vi "Open UI.vi"(8 "error in (no error)":errorcluster, 11 "Process in":refnum<class "Process.lvclass">) -> (0 "error out":errorcluster, 3 "Process out":refnum<class "Process.lvclass">)   [LabVIEW 2021, in "Process.lvlib" / "Process.lvclass"]
uses:
  Process.lvclass
  Process.lvclass/Process.ctl
  LVCAM/Msgs/LVCAM Destroy Self/LVCAM Destroy Self Msg/LVCAM Destroy Self Msg.lvclass
  C:/PPLs/LabVIEW-Composed-Actor-Model-LVCAM/LabVIEW-Composed-Actor-Model-LVCAM/LVCAM/LVCAM/Msg/Msg.lvclass
  LVCAM/LVCAM/Self Actor/Self Msg Send.vi
  LVCAM/LVCAM/Self Actor/Self Actor.lvclass
  C:/PPLs/LabVIEW-Composed-Actor-Model-LVCAM/LabVIEW-Composed-Actor-Model-LVCAM/LVCAM/Msgs/LVCAM Destroy Self/LVCAM Destroy Self Msg/LVCAM Destroy Self Msg.lvclass
  C:/PPLs/LabVIEW-Composed-Actor-Model-LVCAM/LabVIEW-Composed-Actor-Model-LVCAM/LVCAM/Msgs/LVCAM Destroy Self/LVCAM Destroy Self/LVCAM Destroy Self.lvclass
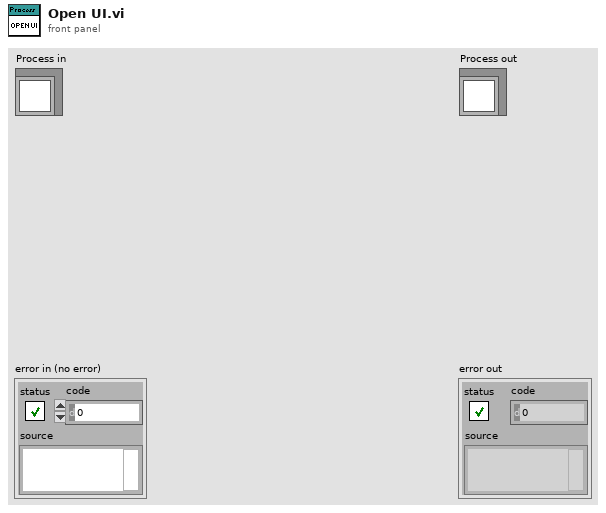
[diagram p1: front panel]
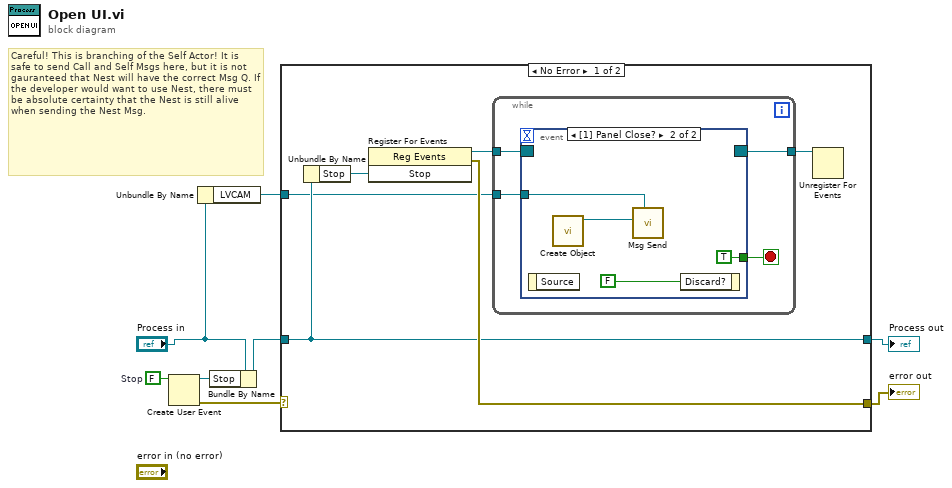
[diagram p0: block diagram]
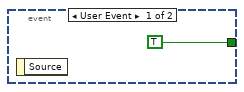
[diagram p2: hidden frame]
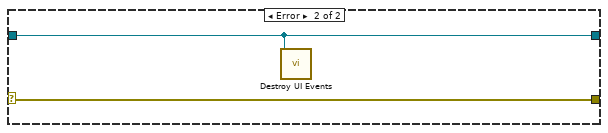
[diagram p3: hidden frame]
diagram:
  w7 = FALSE  # Stop
  # "Careful! This is branching of the Self Actor! It is safe to send Call and Self Msgs here, but it is not gauranteed that Nest will have the correct Msg Q. If the developer would want to use Nest, there must be absolute certainty that the Nest is still alive when sending the Nest Msg."
  n1 = Create User Event(user event datatype=w7) -> (user event=w8:refnum<user-event>, error out=w6:errorcluster)  [unwired: 1 in]
  n2 = Unbundle By Name("Process in") -> ("LVCAM"=w5:refnum<class "LVCAM.lvclass">)
  n3 = Bundle By Name(cluster="Process in", "Stop"=w8) -> (w4:refnum<class "Process.lvclass">)
  n4 = case shown="No Error" w6 {
    selector: w6 -> [_ w25]
    tunnel: [w12 w25] -> w3
    tunnel: w4 -> [w10 w24]
    tunnel: [w10 w24] -> w1
    tunnel: w5 -> [w9 _]
    frame No Error {
      n5 = Unbundle By Name(w10) -> ("Stop"=w11:refnum<user-event>)
      n6 = register-events ("Main Register for Events")(w11) -> (reference out=w14:refnum<event-registration>, error out=w12:errorcluster)  [unwired: 2 in]
      n7 = while {
        tunnel: w14 -> [w18]
        tunnel: [w16] -> w13
        tunnel: w9 -> [w15]
        stop <- w17 stop-if-true
        n8 = event "UI Events" shown="[1] Panel Close?" {
          selector: w18 -> [_ _]
          dyn-events: [_ _] -> w16
          timeout: _ -> [_ _]
          tunnel: [TRUE TRUE] -> w17
          tunnel: w15 -> [_ w23]
          event User Event {
            n9 = event-data() -> ()  [unwired: 1 in, 1 out]
          }
          event Panel Close? {
            n10 = event-data() -> ()  [unwired: 1 in, 1 out]
            n11 = call "Create Object.vi"() -> ("LVCAM Destroy Self Msg out"=w22:refnum<class "LVCAM Destroy Self Msg.lvclass">)  [unwired: 11 in]
            n12 = call-poly "Msg Send.vi"("Self Actor"=w23, "Msg"=w22) -> ()  [unwired: 9 in, 1 out]
            n13 = event-data("Discard?"=FALSE) -> ()  [unwired: 1 in, 1 out]
          }
        }
      }
      n14 = Unregister For Events(event registration refnum=w13) -> ()  [unwired: 1 in, 1 out]
    }
    frame Error {
      n15 = call "Destroy UI Events.vi"("Process in"=w24) -> ()  [unwired: 11 in]
    }
  }
  "error out" <- w3
  "Process out" <- w1
